vi "Insert exchange into jos_content.vi"(2 "Image Name":string, 3 "title":string) -> ()   [LabVIEW 2010]
doc: "This example opens a connection to a database specified by the Connection string (replace the DNS name with your database) inserts a new row into the table \"myOtherTable\" (replace the SQL string with your own SQL query)."
panel:
  out "concatenated string":string
  out "error out":errorcluster
  in  "Command Text":string="INSERT INTO jos_content\n (id, title, alias, introtext, state, sectionid, mask, catid, created_by, modified, modified_by, publish_up, attribs, version, metadesc, metadata)\nVALUES ('id', 'title', 'alias', 'introtext', '1', '14', '0', '1394', '2012-12-12 12:12:12', '62', '2012-12-12 12:12:12', '62', '2012-12-12 12:12:12', 'show_title=\nlink_titles=\nshow_intro=\nshow_section=\nlink_section=\nshow_category=\nlink_category=\nshow_vote=\nshow_author=\nshow_create_date=\nshow_modify_date=\nshow_pdf_icon=\nshow_print_icon=\nshow_email_icon=\nlanguage=\nkeyref=\nreadmore=', '5', 'A book price comparison tool where 2.5% goes towards the cause! | A Student Book Project  Fundraiser', 'robots=\nauthor=');"
  in  "ConnectionString":string="DSN=stusbooks;"
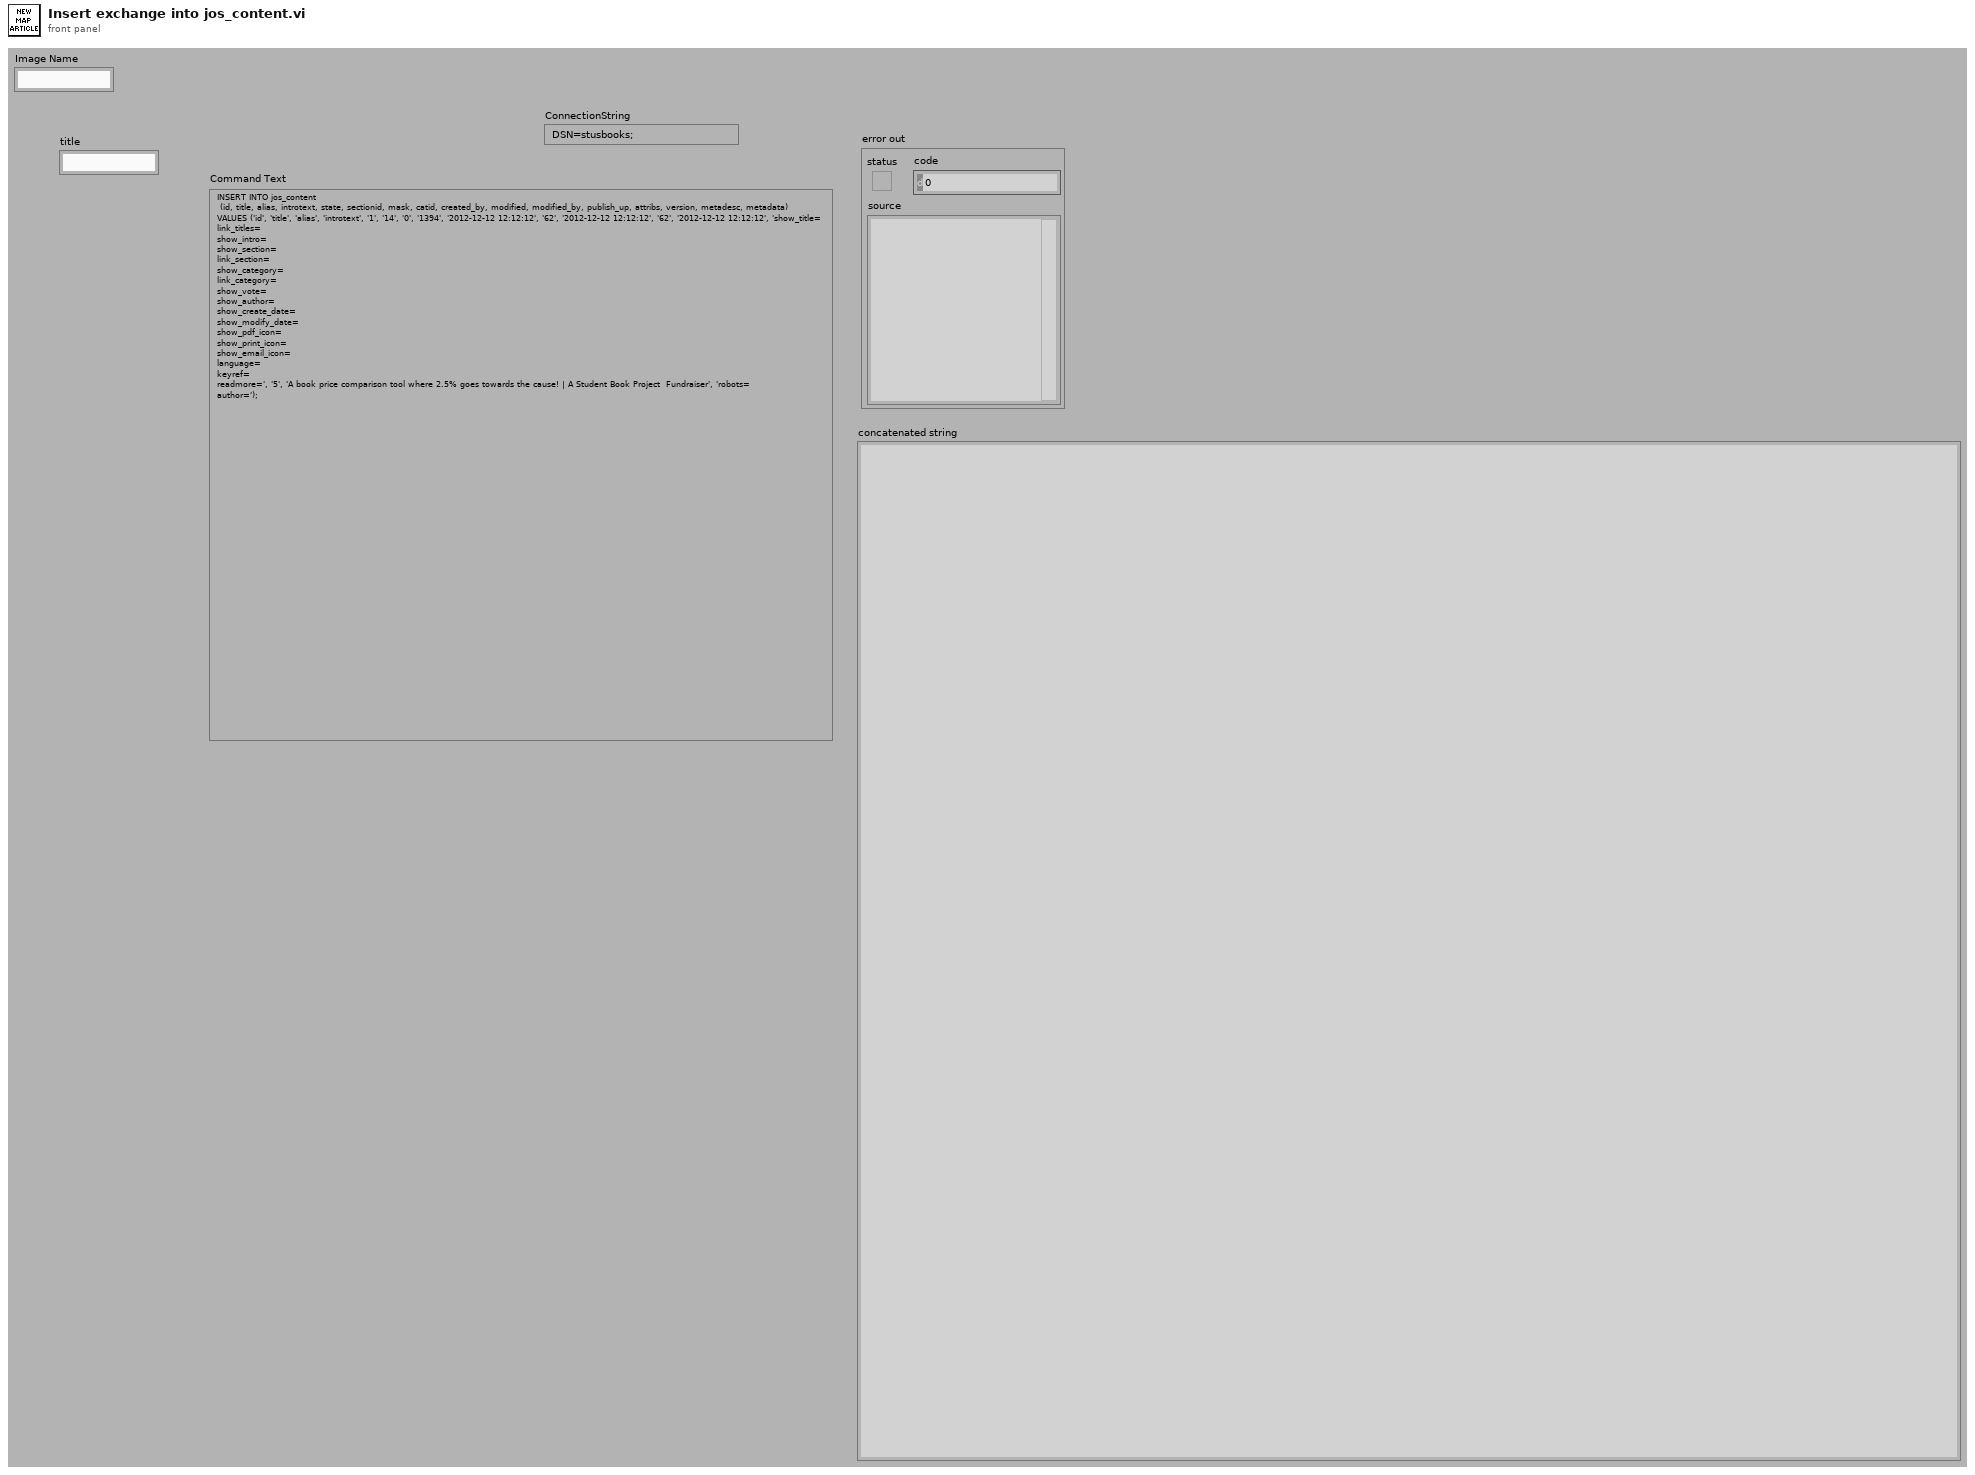
[diagram p1: front panel]
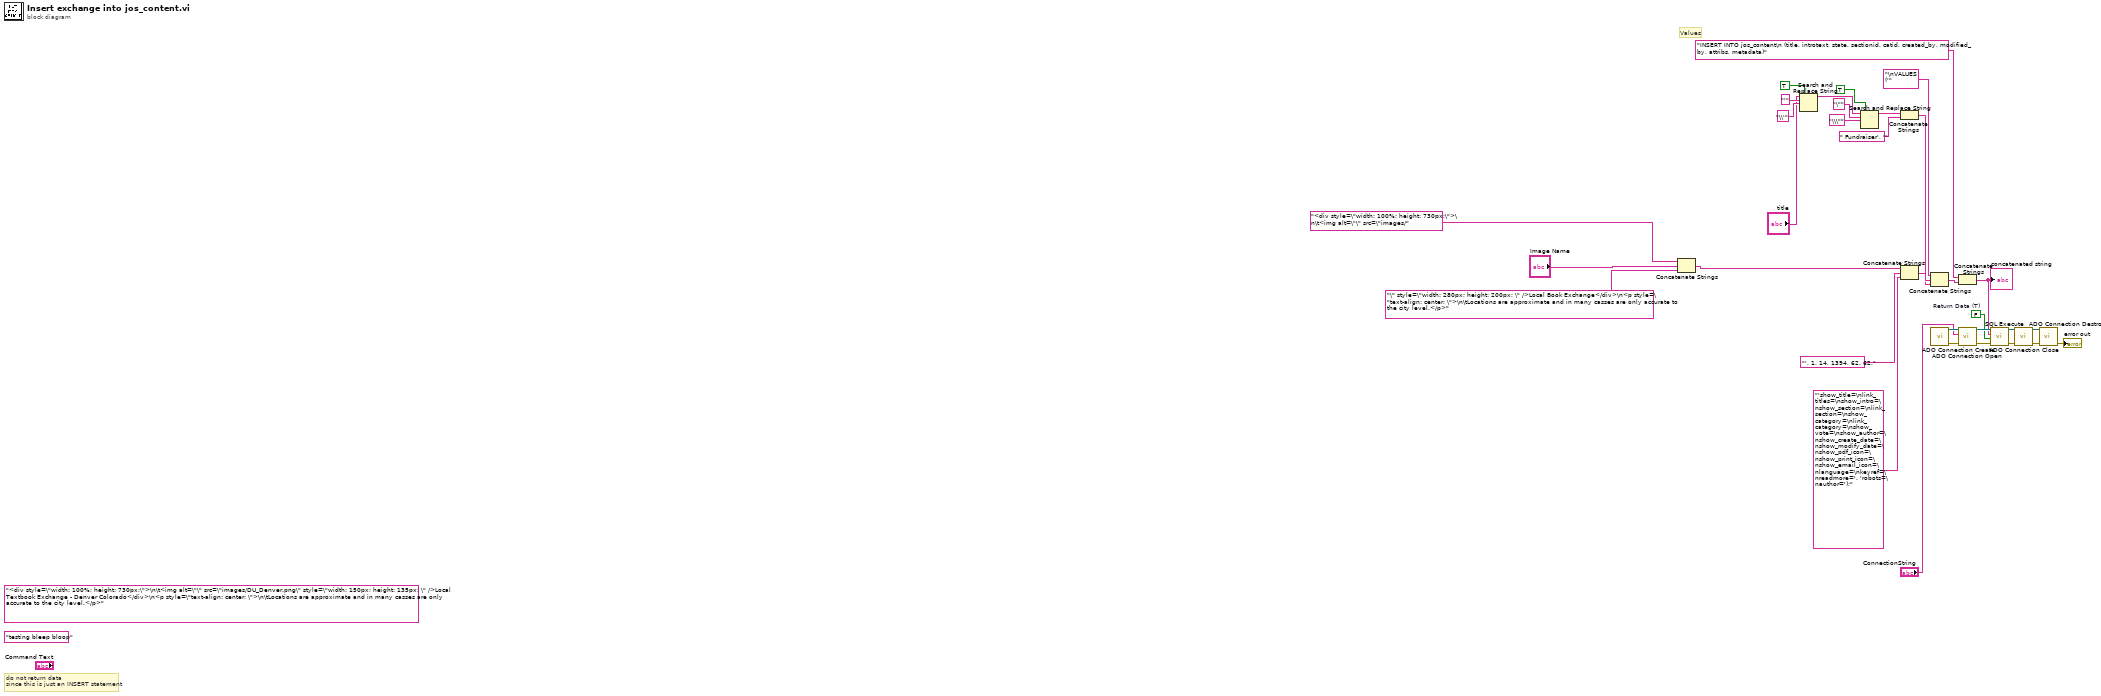
[diagram p0: block diagram]
diagram:
  (unwired) "<div style=\"width: 100%; height: 730px;\">\n\t<img alt=\"\" src=\"images/DU_Denver.png\" style=\"width: 150px; height: 135px; \" />Local Textbook Exchange - Denver Colorado</div>\n<p style=\"text-align: center; \">\n\tLocations are approximate and in many casses are only accurate to the city level.</p>"
  (unwired) "testing bleep bloop"
  w23 = FALSE  # Return Data (T)
  # "Values"
  # "do not return data\nsince this is just an INSERT statement"
  n1 = Concatenate Strings("<div style=\"width: 100%; height: 730px;\">\n\t<img alt=\"\" src=\"images/", "Image Name", "\" style=\"width: 280px; height: 200px; \" />Local Book Exchange</div>\n<p style=\"text-align: center; \">\n\tLocations are approximate and in many casses are only accurate to the city level.</p>" ("string")) -> (w1:string)
  n2 = Search and Replace String(replace all?=TRUE ("replace all? (F)"), input string="title", search string="'", replace string="\\'" ("replace string (\"\")")) -> (result string=w17:string)  [unwired: 4 in, 3 out]
  n3 = Search and Replace String(replace all?=TRUE ("replace all? (F)"), input string=w17, search string="\"", replace string="\\\"" ("replace string (\"\")")) -> (result string=w14:string)  [unwired: 4 in, 3 out]
  n4 = Concatenate Strings(w14, " Fundraiser', '" ("string")) -> (w21:string)
  n5 = Concatenate Strings(w1, "', 1, 14, 1394, 62, 62,", "'show_title=\nlink_titles=\nshow_intro=\nshow_section=\nlink_section=\nshow_category=\nlink_category=\nshow_vote=\nshow_author=\nshow_create_date=\nshow_modify_date=\nshow_pdf_icon=\nshow_print_icon=\nshow_email_icon=\nlanguage=\nkeyref=\nreadmore=', 'robots=\nauthor=');") -> (w7:string)
  n6 = Concatenate Strings("\nVALUES ('" ("string"), w21, w7) -> (w12:string)
  n7 = call "ADO Connection Create.vi"() -> ("error out"=w32:errorcluster, "ADODB._Connection Out"=w33:refnum<k7>)  [unwired: 10 in]
  n8 = call "ADO Connection Open.vi"("error in (no error)"=w32, "ConnectionString"="ConnectionString", "ADODB._Connection In"=w33) -> ("error out"=w29:errorcluster, "ADODB._Connection Out"=w30:refnum<k7>)  [unwired: 7 in]
  n9 = Concatenate Strings("INSERT INTO jos_content\n (title, introtext, state, sectionid, catid, created_by, modified_by, attribs, metadata)" ("string"), w12) -> (w10:string)
  "concatenated string" <- w10
  n10 = call "SQL Execute.vi"("error in (no error)"=w29, "Return Data (T)"=w23, "Command Text"=w10, "ADODB._Connection In"=w30) -> ("error out"=w28:errorcluster, "ADODB._Connection Out"=w27:refnum<k7>)  [unwired: 4 in, 2 out]
  n11 = call "ADO Connection Close.vi"("error in (no error)"=w28, "ADODB._Connection In"=w27) -> ("error out"=w26:errorcluster, "ADODB._Connection Out"=w25:refnum<k7>)  [unwired: 8 in]
  n12 = call "ADO Connection Destroy.vi"("error in (no error)"=w26, "ADODB._Connection In"=w25) -> ("error out"=→"error out":errorcluster)  [unwired: 9 in]
